vi "习题3.2.vi"() -> ()   [LabVIEW 2017]
panel:
  out "数值 3":dbl
  in  "数值 2":dbl
  in  "数值":dbl
  in  "枚举":enum16{"加法", "减法", "乘法", "除法"}(ring)
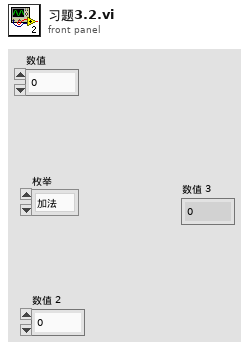
[diagram p1: front panel]
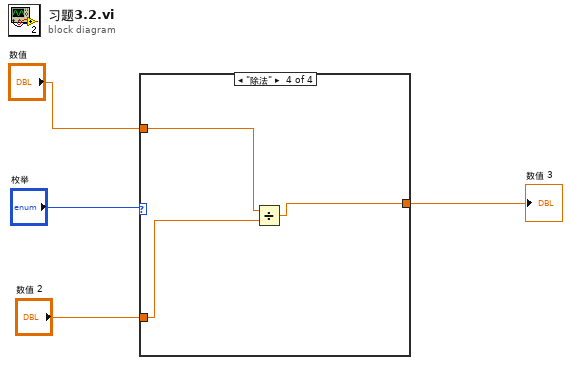
[diagram p0: block diagram]
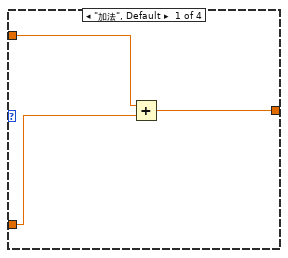
[diagram p2: hidden frame]
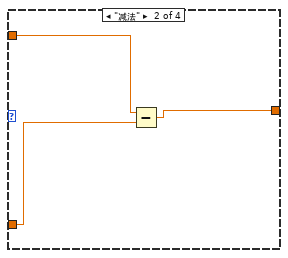
[diagram p3: hidden frame]
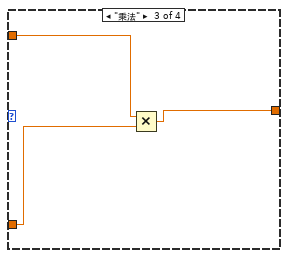
[diagram p4: hidden frame]
diagram:
  n1 = case shown="\"除法\"" "枚举" {
    tunnel: "数值 2" -> [w6 w9 w12 w15]
    tunnel: "数值" -> [w7 w10 w13 w16]
    tunnel: [w5 w8 w11 w14] -> w1
    frame "加法", Default {
      n2 = Add(x=w7, y=w6) -> (x+y=w5:dbl)
    }
    frame "减法" {
      n3 = Subtract(x=w10, y=w9) -> (x-y=w8:dbl)
    }
    frame "乘法" {
      n4 = Multiply(x=w13, y=w12) -> (x*y=w11:dbl)
    }
    frame "除法" {
      n5 = Divide(x=w16, y=w15) -> (x/y=w14:dbl)
    }
  }
  "数值 3" <- w1
